vi "ConvertGoop3ToGoop4_ReplaceGetAttToModify.vi"(8 "error in (no error)":errorcluster, 9 "GetClassAttributeVI":path, 10 "GetAttributeVI":path, 11 "ViRef":refnum<vi>) -> (0 "error out":errorcluster, 3 "ViRefOut":refnum<vi>)   [LabVIEW 2016]
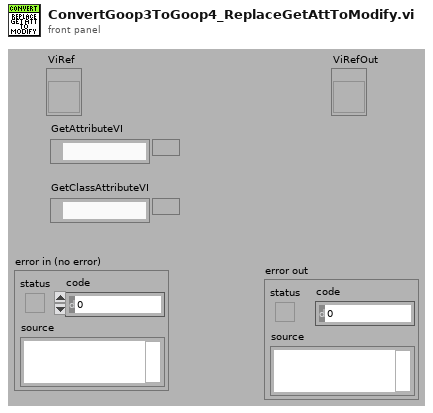
[diagram p1: front panel]
types:
  T1 = enum32{"invalid lock state", "Not Locked", "Locked (No Password)", "Password-protected"}
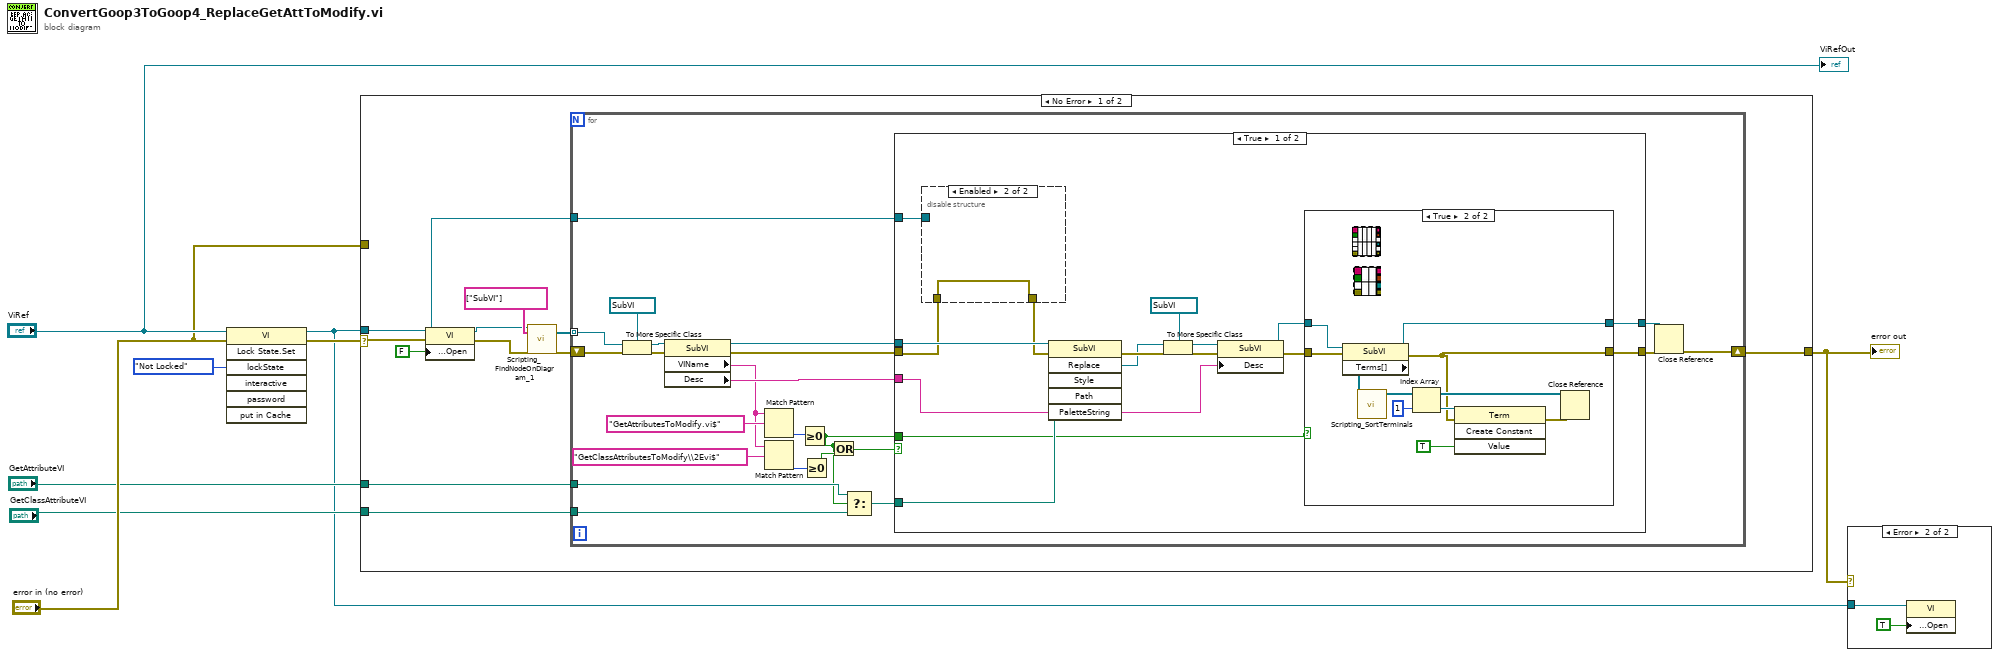
[diagram p0: block diagram]
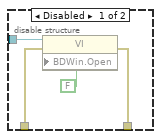
[diagram p3: hidden frame]
diagram:
  n1 = invoke class="VI" method="Lock State.Set"(reference="ViRef", error in="error in (no error)", "lockState"=T1."Not Locked" ("Lock State")) -> (reference out=w1:refnum<vi>, error out=w6:errorcluster)  [unwired: 4 in, 5 out]
  n2 = case shown="No Error" w6 {
    selector: w6 -> [w12 _]
    tunnel: [w14 w78] -> w2
    tunnel: w1 -> [w9 _]
    tunnel: "error in (no error)" -> [_ w78]
    tunnel: "GetAttributeVI" -> [w11 _]
    tunnel: "GetClassAttributeVI" -> [w10 _]
    frame No Error {
      n3 = property class="VI"(reference=w9, error in=w12, "Front Panel.Open"=FALSE ("Front Panel Window:Open")) -> (reference out=w16:refnum<vi>, error out=w13:errorcluster)
      n4 = call <resource>:"Scripting_FindNodeOnDiagram_1.vi"("ViRef(Ignored If Not Wired)"=w16, "NodeTypesToSearchFor"=string[] ["SubVI"], "error in (no error)"=w13) -> ("Nodes"=w18:refnum<vi>[], "error out"=w17:errorcluster)  [unwired: 15 in]
      n5 = for {
        tunnel: w18 -> [w42] mode=indexing
        shift-right: [w34] -> w14
        shift-left: w17 -> [w40]
        tunnel: w11 -> [w24]
        tunnel: w10 -> [w22]
        tunnel: w9 -> [w20]
        n6 = To More Specific Class(target class=refnum<vi> refnum ("WhileLoop"), reference=w42, error in=w40) -> (specific class reference=w39:refnum<vi>, error out=w38:errorcluster)
        n7 = property class="SubVI"(reference=w39, error in=w38) -> (reference out=w37:refnum<vi>, error out=w36:errorcluster, "VIName"=w29:string, "Desc"=w30:string)
        n8 = Match Pattern(string=w29, regular expression="GetAttributesToModify.vi$") -> (offset past match=w31:i32)  [unwired: 1 in, 3 out]
        n9 = Match Pattern(string=w29, regular expression="GetClassAttributesToModify\\2Evi$") -> (offset past match=w27:i32)  [unwired: 1 in, 3 out]
        n10 = Greater Or Equal To 0?(x=w31) -> (x >= 0?=w21:bool)
        n11 = Greater Or Equal To 0?(x=w27) -> (x >= 0?=w25:bool)
        n12 = Or(x=w21, y=w25) -> (x .or. y?=w26:bool)
        n13 = Select(t=w24, s=w21, f=w22) -> (s? t:f=w23:path)
        n14 = case shown="True" w26 {
          tunnel: w37 -> [w58 w76]
          tunnel: w36 -> [w44 w77]
          tunnel: [w48 w77] -> w35
          tunnel: [w47 w76] -> w33
          tunnel: w23 -> [w57 _]
          tunnel: w30 -> [w51 _]
          tunnel: w21 -> [w50 _]
          tunnel: w20 -> [w45 _]
          frame True {
            n15 = disable-structure shown="Enabled" {
              disable-tunnel: w45 -> [w61 _]
              disable-tunnel: w44 -> [w60 w63]
              disable-tunnel: [w59 w63] -> w43
              frame Disabled {
                n16 = property class="VI"(reference=w61, error in=w60, "BDWin.Open"=FALSE ("Front Panel Window:Open")) -> (error out=w59:errorcluster)  [unwired: 1 out]
              }
              frame Enabled {
              }
            }
            n17 = invoke class="SubVI" method="Replace"(reference=w58, error in=w43, "Path"=w57) -> (error out=w55:errorcluster, "Replace"=w52:refnum<vi>)  [unwired: 3 in, 4 out]
            n18 = To More Specific Class(target class=refnum<vi> refnum ("WhileLoop"), reference=w52, error in=w55) -> (specific class reference=w53:refnum<vi>, error out=w54:errorcluster)
            n19 = property class="SubVI"(reference=w53, error in=w54, "Desc"=w51) -> (reference out=w46:refnum<vi>, error out=w49:errorcluster)
            n20 = case shown="True" w50 {
              tunnel: w49 -> [w65 w75]
              tunnel: [w65 w66] -> w48
              tunnel: [w64 w69] -> w47
              tunnel: w46 -> [w64 w74]
              frame False {
              }
              frame True {
                n21 = property class="SubVI"(reference=w74, error in=w75) -> (reference out=w69:refnum<vi>, error out=w66:errorcluster, "Terms[]"=w73:refnum<vi>[])
                n22 = call <resource>:"Scripting_SortTerminals.vi"("Terminals[]"=w73) -> ("TerminalsOut[]"=w67:refnum<vi>[])  [unwired: 8 in, 2 out]
                n23 = Index Array(array=w67, index=1) -> (element=w71:refnum<vi>)
                n24 = invoke class="Term" method="Create Constant"(reference=w71, error in=w66, "Value"=TRUE) -> (error out=w68:errorcluster)  [unwired: 1 in, 3 out]
                n25 = Close Reference(reference=w67, error in (no error)=w68) -> ()  [unwired: 1 out]
              }
            }
          }
          frame False {
          }
        }
        n26 = Close Reference(reference=w33, error in (no error)=w35) -> (error out=w34:errorcluster)
      }
    }
    frame Error {
    }
  }
  "error out" <- w2
  n27 = case shown="Error" w2 {
    tunnel: w1 -> [_ w79]
    frame No Error {
    }
    frame Error {
      n28 = property class="VI"(reference=w79, "Front Panel.Open"=TRUE ("Front Panel Window:Open")) -> ()  [unwired: 1 in, 2 out]
    }
  }
  "ViRefOut" <- "ViRef"
